vi "Preset SOFT. AGC.vi"(8 "error in (no error)":errorcluster, 10 "on/off":u16(ring) items=["OFF", "ON"], 11 "VISA resource in":refnum<visa-resource-name>) -> (0 "error out":errorcluster, 3 "VISA resource out":refnum<visa-resource-name>)   [LabVIEW 2025, in "Chroma 19572.lvlib"]
doc: "This VI writes to the instrument the SOFT. AGC state."
uses:
  <instrlib>/Chroma 19572/Chroma 19572.lvlib
panel:
  # "PreSet SOFT. AGC (Automatic Gain Compensation)"
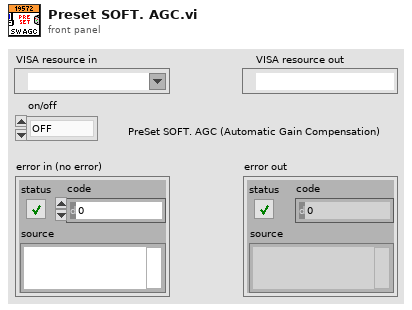
[diagram p1: front panel]
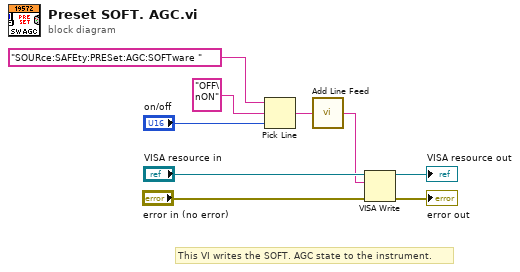
[diagram p0: block diagram]
diagram:
  # "This VI writes the SOFT. AGC state to the instrument."
  n1 = Pick Line(string ("")="SOURce:SAFEty:PRESet:AGC:SOFTware ", multi-line string="OFF\nON", line index="on/off") -> (output string=w2:string)
  n2 = call <instrlib>:"Add Line Feed.vi"("Command string"=w2) -> ("Concatenated string"=w1:string)  [unwired: 4 in]
  n3 = VISA Write(VISA resource name="VISA resource in", write buffer=w1, error in (no error)="error in (no error)") -> (VISA resource name out=→"VISA resource out":refnum<visa-resource-name>, error out=→"error out":errorcluster)  [unwired: 1 out]
